vi "DAQ_Mode.vi"() -> ()   [LabVIEW 2013]
panel:
  out "DAQ mode?":bool
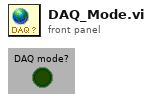
[diagram p1: front panel]
diagram:
